vi "Update Component.vi"(8 "error in (no error)":errorcluster, 10 "Component":T1, 11 "Blueprint in":refnum<class "Blueprint.lvclass">) -> (0 "error out":errorcluster, 3 "Blueprint out":refnum<class "Blueprint.lvclass">)   [LabVIEW 2020, in "Blueprint.lvclass"]
uses:
  Blueprint.lvclass
  Item/Ingredient.ctl
  Item/Item.lvclass
  Blueprint.lvclass/Blueprint.ctl
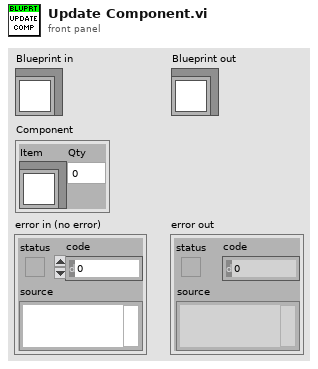
[diagram p1: front panel]
types:
  T1 = typedef "Item.lvclass/Ingredient.ctl" = cluster{"Item":refnum<class "Item.lvclass">, "Qty":dbl}
  T2 = typedef "Blueprint.lvclass/Ref Data.ctl" = cluster{"Ingredients":T1[], "Workstation":refnum<class "Workstation.lvclass">, "Craft Time":dbl, "Name":string}
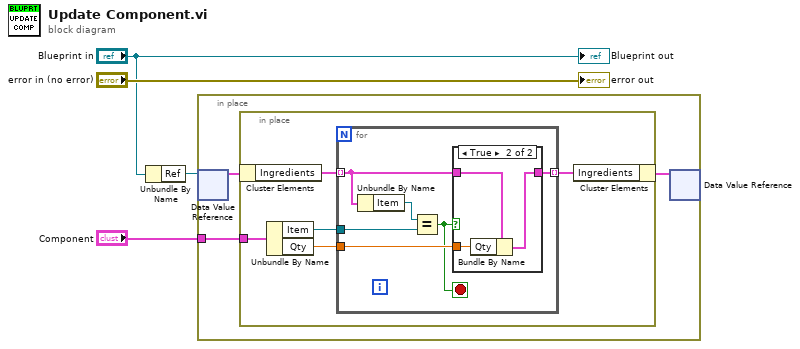
[diagram p0: block diagram]
diagram:
  n1 = Unbundle By Name("Blueprint in") -> ("Ref"=w3:refnum<data-value>)
  n2 = in-place {
    in-place-border: "Component" -> [w5]
    n3 = in-place-dvr #1(w3) -> (w7:T2)  [unwired: 1 out]
    n4 = in-place {
      in-place-border: w5 -> [w11]
      n5 = in-place-cluster #2(w7) -> ("Ingredients"=w12:T1[])
      n6 = Unbundle By Name(w11) -> ("Item"=w10:refnum<class "Item.lvclass">, "Qty"=w9:dbl)
      n7 = for {
        tunnel: w12 -> [w16] mode=indexing
        tunnel: w10 -> [w18]
        tunnel: w9 -> [w15]
        tunnel: [w14] -> w8 mode=indexing
        stop <- w13 stop-if-true
        n8 = Unbundle By Name(w16) -> ("Item"=w17:refnum<class "Item.lvclass">)
        n9 = Equal?(x=w17, y=w18) -> (x = y?=w13:bool)
        n10 = case shown="True" w13 {
          tunnel: w16 -> [w19 w22]
          tunnel: w15 -> [_ w21]
          tunnel: [w19 w20] -> w14
          frame False {
          }
          frame True {
            n11 = Bundle By Name(cluster=w22, "Qty"=w21) -> (w20:T1)
          }
        }
      }
      n12 = in-place-cluster #2("Ingredients"=w8) -> (w6:T2)
    }
    n13 = in-place-dvr #1(w6) -> ()  [unwired: 2 out]
  }
  "error out" <- "error in (no error)"
  "Blueprint out" <- "Blueprint in"
